vi "Example-Uart.vi"() -> ()   [LabVIEW 2018]
uses:
  c8864175-e948-409a-9e2f-56297bfabe3e.vi
panel:
  in  "Read":bool
  in  "Write":bool=TRUE
  in  "loop":i32=100
  out "数值":i32
  out "波形图":u8[](graph)
  out "SerialNumber":string
  out "rxcount out":i32
  out "rgRX":u8[](array[numeric])
  in  "Tx data":u8[](array[numeric])=[1, 2, 3, 4, 5]
  in  "RX IO(0~15)":i32=1
  in  "TX IO(0~15)":i32
  in  "Frequency(Hz)":i32(ring)=9600 items=["110"=110, "150"=150, "300"=300, "600"=600, "1200"=1200, "2400"=2400, "4800"=4800, "9600"=9600, "14400"=14400, "19200"=19200, "28800"=28800, "38400"=38400, "56000"=56000, "57600"=57600, "115200"=115200, "128000"=128000, "153600"=153600, "230400"=230400, "256000"=256000, "406800"=406800, "921600"=921600]
  out "returns":i32[](array[numeric])
  out "error out":errorcluster caption="错误输出"
  in  "error in (no error)":errorcluster caption="错误输入（无错误）"
  out "ftHandle out":u64=363562184
  in  "设备索引":i32=1
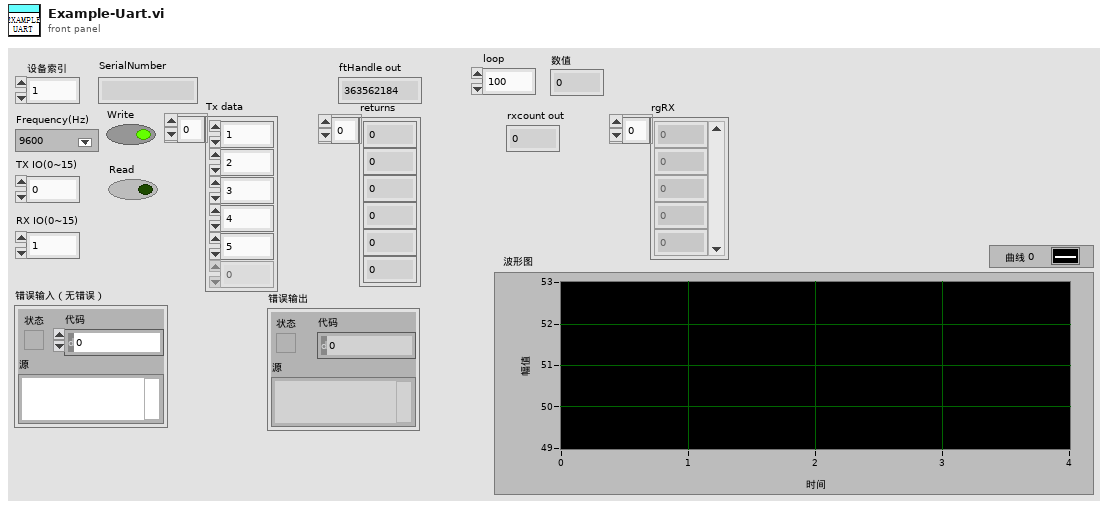
[diagram p1: front panel]
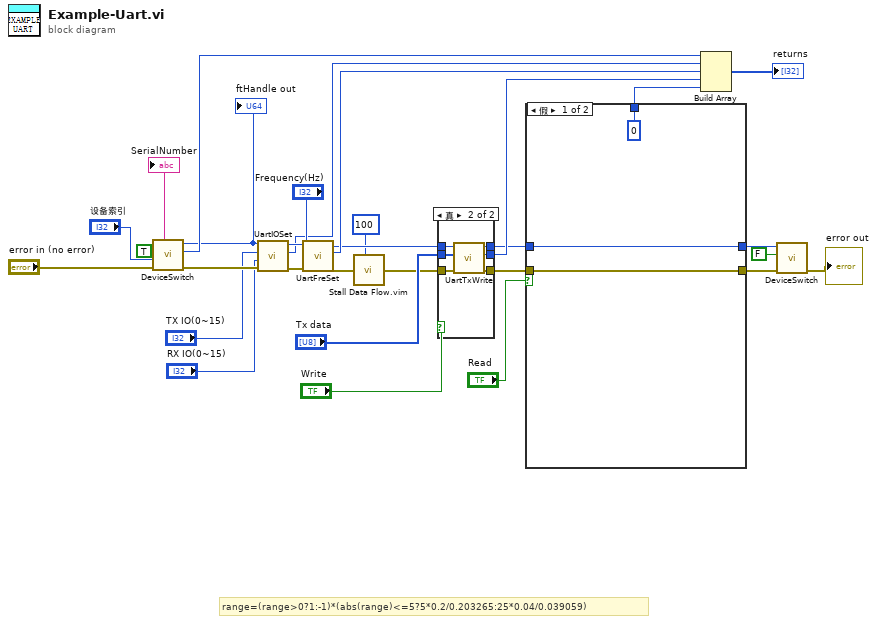
[diagram p0: block diagram]
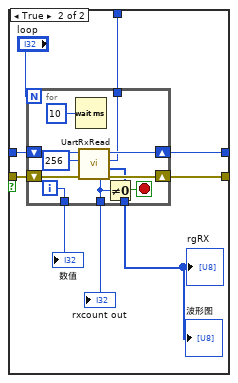
[diagram p2: hidden frame]
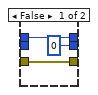
[diagram p3: hidden frame]
diagram:
  # "range=(range>0?1:-1)*(abs(range)<=5?5*0.2/0.203265:25*0.04/0.039059)"
  n1 = call "DeviceSwitch.vi"("error in (no error)"="error in (no error)", "Device Index"="设备索引", "Open"=TRUE) -> ("error out"=w25:errorcluster, "function return"=w26:i32, "handle out"=w3:u64, "SerialNumber"=→"SerialNumber":string)  [unwired: 4 in, 1 out]
  "ftHandle out" <- w3
  n2 = call "UartIOSet.vi"("error in (no error)"=w25, "RX IO(0~15)"="RX IO(0~15)", "TX IO(0~15)"="TX IO(0~15)", "handle"=w3) -> ("error out"=w24:errorcluster, "function return"=w19:i32, "handle out"=w20:u64)  [unwired: 5 in]
  n3 = call "UartFreSet.vi"("error in (no error)"=w24, "Frequency(Hz)"="Frequency(Hz)", "handle"=w20) -> ("error out"=w15:errorcluster, "function return"=w18:i32, "handle out"=w17:u64)  [unwired: 6 in]
  n4 = call "Stall Data Flow.vim"("value in"=w15, "milliseconds to wait"=u32 100) -> ("value out"=w2:errorcluster)  [unwired: 1 out]
  n5 = case shown="真" "Write" {
    tunnel: w17 -> [w33 w39]
    tunnel: "Tx data" -> [_ w38]
    tunnel: w2 -> [w31 w37]
    tunnel: [0 ("function return") w36] -> w14
    tunnel: [w31 w35] -> w7
    tunnel: [w33 w34] -> w6
    frame False {
    }
    frame True {
      n6 = call "UartTxWrite.vi"("error in (no error)"=w37, "data"=w38, "handle"=w39) -> ("error out"=w35:errorcluster, "function return"=w36:i32, "handle out"=w34:u64)  [unwired: 6 in]
    }
  }
  n7 = case shown="假" "Read" {
    tunnel: [0 ("function return") w51] -> w13
    tunnel: [w41 w50] -> w9
    tunnel: [w42 w49] -> w8
    tunnel: w7 -> [w41 w48]
    tunnel: w6 -> [w42 w47]
    frame False {
    }
    frame True {
      n8 = for {
        N: "loop" -> [_]
        tunnel: [w58] -> w51
        tunnel: [w57] -> w44
        tunnel: [w56] -> w46
        shift-right: [w61] -> w50
        shift-left: w48 -> [w62]
        shift-right: [w60] -> w49
        shift-left: w47 -> [w59]
        tunnel: [w53] -> w43
        i -> [w53]
        stop <- w55 stop-if-true
        n9 = Wait (ms)(milliseconds to wait=u32 10 ("等待时间（毫秒）")) -> ()  [unwired: 1 out]
        n10 = call "UartRxRead.vi"("error in (no error)"=w62, "length"=256, "handle"=w59) -> ("error out"=w61:errorcluster, "rgRX"=w57:u8[], "function return"=w58:i32, "handle out"=w60:u64, "rxcount out"=w56:i32)  [unwired: 4 in]
        n11 = Not Equal To 0?(x=w56) -> (x != 0?=w55:bool)
      }
      "rgRX" <- w44
      "rxcount out" <- w46
      "波形图" <- w44
      "数值" <- w43
    }
  }
  n12 = Build Array(w26, w19, w18, w14, w13) -> (→"returns":i32[])
  n13 = call "DeviceSwitch.vi"("error in (no error)"=w9, "Open"=FALSE, "handle"=w8) -> ("error out"=→"error out":errorcluster)  [unwired: 4 in, 4 out]
